vi "Configure Current Channel Trigger.vi"(6 "Trigger Count (1)":i32=1, 7 "Trigger Mode (0: Channel)":i32(ring) items=["Channel", "Sweep", "Point", "Trace"], 8 "error in (no error)":errorcluster, 9 "Trigger Condition (1: Continuous)":i32(ring)=1 items=["Hold", "Continuous", "Groups", "Single"], 10 "Channel (1)":i32=1, 11 "VISA resource name":refnum<visa-resource-name>) -> (0 "error out":errorcluster, 3 "VISA resource name out":refnum<visa-resource-name>)   [LabVIEW 2018, in "Keysight PNA Series.lvlib"]
doc: "Configures the trigger of current channel."
uses:
  Keysight PNA Series.lvlib
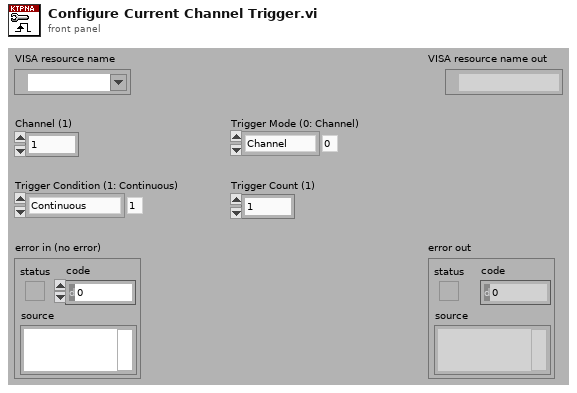
[diagram p1: front panel]
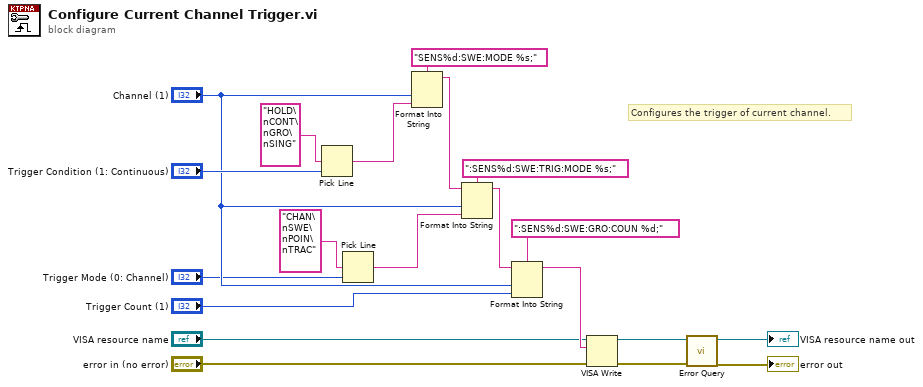
[diagram p0: block diagram]
diagram:
  # "Configures the trigger of current channel."
  n1 = Pick Line(multi-line string="HOLD\nCONT\nGRO\nSING", line index="Trigger Condition (1: Continuous)") -> (output string=w16:string)  [unwired: 1 in]
  n2 = Pick Line(multi-line string="CHAN\nSWE\nPOIN\nTRAC", line index="Trigger Mode (0: Channel)") -> (output string=w11:string)  [unwired: 1 in]
  n3 = Format Into String(format string="SENS%d:SWE:MODE %s;", "Channel (1)", w16) -> (resulting string=w13:string)  [unwired: 2 in, 1 out]
  n4 = Format Into String(format string=":SENS%d:SWE:TRIG:MODE %s;", initial string=w13, "Channel (1)", w11) -> (resulting string=w10:string)  [unwired: 1 in, 1 out]
  n5 = Format Into String(format string=":SENS%d:SWE:GRO:COUN %d;", initial string=w10, "Channel (1)", "Trigger Count (1)") -> (resulting string=w7:string)  [unwired: 1 in, 1 out]
  n6 = VISA Write(VISA resource name="VISA resource name", write buffer=w7, error in (no error)="error in (no error)") -> (VISA resource name out=w4:refnum<visa-resource-name>, error out=w3:errorcluster)  [unwired: 1 out]
  n7 = call "Error Query.vi"("error in (no error)"=w3, "VISA resource name"=w4) -> ("error out"=→"error out":errorcluster, "VISA resource name out"=→"VISA resource name out":refnum<visa-resource-name>)  [unwired: 6 in, 2 out]
